vi "Begin.vi"(8 "error in":errorcluster) -> (0 "error out":errorcluster)   [LabVIEW 2016]
doc: "Called before other user functions, this VI is expected to open initial I/O refnums, load in file data, and do all program initialization. Notice that the <B>error out</B> terminal is simply used for data flow. Wiring it to other structures or subVIs ensures that this VI runs first."
uses:
  <vilib>/Rock Robotics/SystemInterfaces/DIO/FPGA_DIOPWMChannel.ctl
  <vilib>/Rock Robotics/WPI/SafetyOutput/WPI_SafetyOutputConfigMenu.ctl
  <vilib>/Rock Robotics/WPI/DriverStation/WPI_DriverStationRobotMode2.ctl
  <vilib>/Rock Robotics/WPI/Joystick/WPI_JoystickDeviceEnum.ctl
  <vilib>/Rock Robotics/SystemInterfaces/DIO/FPGA_DIOChannel.ctl
  <vilib>/Rock Robotics/SystemInterfaces/AI/FPGA_AIChannel.ctl
  <vilib>/Rock Robotics/WPI/RobotDrive/WPI_RobotDriveOpen2MotorWithVictorSP.vi
  Robot Global Data.vi
  <vilib>/Rock Robotics/Network Tables/NT Write String Array.vi
  <vilib>/Rock Robotics/WPI/MotorControl/WPI_MotorControlOpen VictorSP.vi
  <vilib>/Rock Robotics/WPI/Switch/WPI_SwitchOpenLimit.vi
  <vilib>/Rock Robotics/WPI/Counter/WPI_CounterDigitalInputToDigitalSource.vi
  <vilib>/Rock Robotics/WPI/Counter/WPI_CounterOpen UpDown Mode.vi
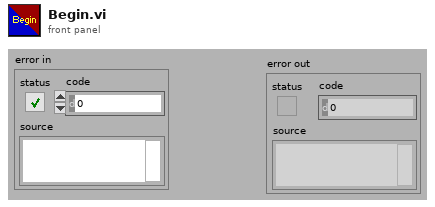
[diagram p1: front panel]
types:
  T1 = typedef "FPGA_DIOChannel.ctl" = enum8{"DIO 0", "DIO 1", "DIO 2", "DIO 3", "DIO 4", "DIO 5", "DIO 6", "DIO 7", "DIO 8", "DIO 9", "DIO MXP 0", "DIO MXP 1", "DIO MXP 2", "DIO MXP 3", "DIO MXP 4", "DIO MXP 5", "DIO MXP 6", "DIO MXP 7", "DIO MXP 8", "DIO MXP 9", "DIO MXP 10", "DIO MXP 11", "DIO MXP 12", "DIO MXP 13", "DIO MXP 14", "DIO MXP 15", "SPI Port CS1", "SPI Port CS2", "SPI Port CS3", "SPI Port MISO", "SPI Port MOSI", "Invalid"}
  T2 = typedef "FPGA_AIChannel.ctl" = enum8{"AI 0", "AI 1", "AI 2", "AI 3", "AI MXP 0", "AI MXP 1", "AI MXP 2", "AI MXP 3", "Invalid"}
  T3 = typedef "FPGA_DIOPWMChannel.ctl" = enum8{"PWM 0", "PWM 1", "PWM 2", "PWM 3", "PWM 4", "PWM 5", "PWM 6", "PWM 7", "PWM 8", "PWM 9", "PWM MXP 0", "PWM MXP 1", "PWM MXP 2", "PWM MXP 3", "PWM MXP 4", "PWM MXP 5", "PWM MXP 6", "PWM MXP 7", "PWM MXP 8", "PWM MXP 9", "Invalid"}
  T4 = typedef "WPI_JoystickDeviceEnum.ctl" = enum16{"USB 0", "USB 1", "USB 2", "USB 3", "USB 4", "USB 5"}
  T5 = typedef "WPI_DriverStationRobotMode2.ctl" = enum16{"Autonomous Disabled", "Autonomous Enabled", "Teleop Disabled", "Teleop Enabled", "Disconnected", "Finish", "Test Disabled", "Test Enabled", "Emergency Stopped"}
  T6 = typedef "WPI_SafetyOutputConfigMenu.ctl" = enum16{"Enable", "Disable"}
  T7 = typedef "WPI_MotorControlDeviceRef.ctl" = cluster{"DeviceStatus":errorcluster, "Type":T8, "PWM":cluster{"PWM Channel":T3, "DeadBand":T9}, "CAN":cluster{"Device Number":u8, "SetOutput VI Ref":variant, "GetOutput VI Ref":variant, "Enable VI Ref":variant, "Disable VI Ref":variant, "Data":variant}, "Invert":bool}
  T8 = typedef "WPI_MotorControlType.ctl" = enum16{"PWM", "CAN"}
  T9 = typedef "WPI_PWMDeadband.ctl" = cluster{"Name":string, "maxPositivePwm":i32, "minPositivePwm":i32, "centerPwm":i32, "maxNegativePwm":i32, "minNegativePwm":i32, "angularRange":u16}
  T10 = typedef "WPI_RobotDriveDevRef.ctl" = cluster{"DevStatus":errorcluster, "Motors[]":T7[], "Square Inputs":bool, "Max Output":dbl}
  T11 = typedef "WPI_JoystickDevRef.ctl" = cluster{"Device":T4}
  T12 = typedef "WPI_ServoDeviceRef.ctl" = cluster{"DeviceStatus":errorcluster, "PWM Channel":T3, "DeadBand":T9}
  T13 = typedef "WPI_SwitchDevRef.ctl" = cluster{"DevStatus":errorcluster, "DIO Channel":T1, "CntIndex":T14, "Normally Closed":bool}
  T14 = typedef "FPGA_CounterCtrSystemIndex.ctl" = enum8{"Ctr 0", "Ctr 1", "Ctr 2", "Ctr 3", "Ctr 4", "Ctr 5", "Ctr 6", "Ctr 7", "Invalid"}
  T15 = typedef "WPI_PotentiometerDevRef.ctl" = cluster{"DevStatus":errorcluster, "Analog Channel":T2, "Invert Output":bool}
  T16 = typedef "WPI_DigitalInputDevRef.ctl" = cluster{"DevStatus":errorcluster, "DIO Channel":T1}
  T17 = typedef "FPGA_CounterEncoderSourceConvertionLVSourceType.ctl" = cluster{"DevStatus":errorcluster, "AnalogTriggerMode?":bool, "DigitalMode":cluster{"DIO Channel":T18}, "AnalogTriggerMode":cluster{"AnalogTriggerIndex":T19, "OutputType":T20}}
  T18 = typedef "FPGA_DIODigitalSourceChannel.ctl" = enum8{"DIO 0", "DIO 1", "DIO 2", "DIO 3", "DIO 4", "DIO 5", "DIO 6", "DIO 7", "DIO 8", "DIO 9", "DIO MXP 0", "DIO MXP 1", "DIO MXP 2", "DIO MXP 3", "DIO MXP 4", "DIO MXP 5", "DIO MXP 6", "DIO MXP 7", "DIO MXP 8", "DIO MXP 9", "DIO MXP 10", "DIO MXP 11", "DIO MXP 12", "DIO MXP 13", "DIO MXP 14", "DIO MXP 15", "Disabled"}
  T19 = typedef "FPGA_AnalogTriggerIndex.ctl" = enum8{"Trig 0", "Trig 1", "Trig 2", "Trig 3", "Trig 4", "Trig 5", "Trig 6", "Trig 7", "Invalid"}
  T20 = typedef "FPGA_AnalogTriggerOutType.ctl" = enum16{"InWindow", "TriggerState", "Rising", "Falling"}
  T21 = typedef "WPI_CounterDevRef.ctl" = cluster{"DevStatus":errorcluster, "CntIndex":T14}
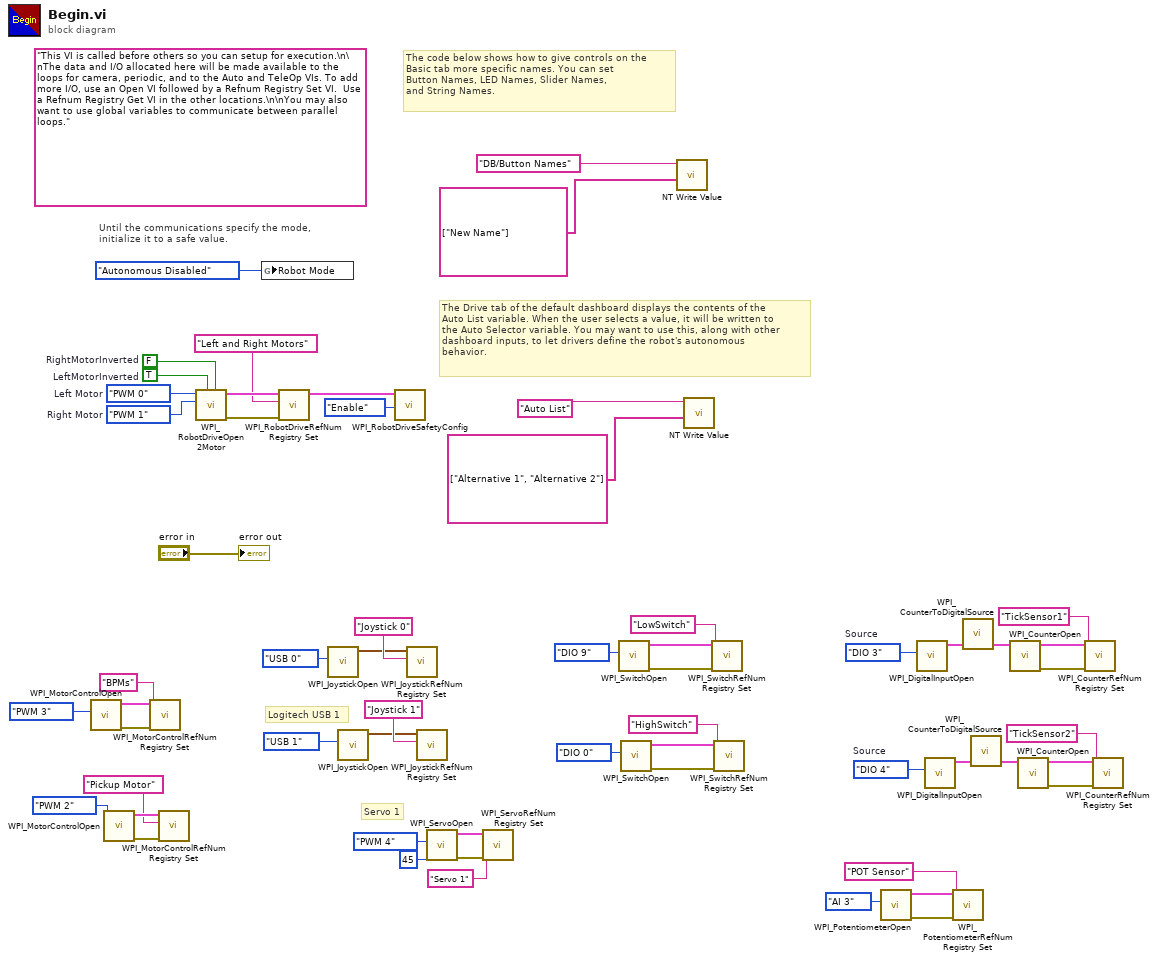
[diagram p0: block diagram]
diagram:
  w5 = FPGA_DIOChannel."DIO 4"  # Source
  w11 = FPGA_DIOChannel."DIO 3"  # Source
  (unwired) "This VI is called before others so you can setup for execution.\n\nThe data and I/O allocated here will be made available to the loops for camera, periodic, and to the Auto and TeleOp VIs. To add more I/O, use an Open VI followed by a Refnum Registry Set VI.  Use a Refnum Registry Get VI in the other locations.\n\nYou may also want to use global variables to communicate between parallel loops."
  w52 = FPGA_DIOPWMChannel."PWM 1"  # Right Motor
  w53 = FPGA_DIOPWMChannel."PWM 0"  # Left Motor
  w57 = TRUE  # LeftMotorInverted
  w58 = FALSE  # RightMotorInverted
  # "Logitech USB 1"
  # "Servo 1"
  # "The Drive tab of the default dashboard displays the contents of the\nAuto List variable. When the user selects a value, it will be written to\nthe Auto Selector variable. You may want to use this, along with other\ndashboard inputs, to let drivers define the robot's autonomous\nbehavior."
  # "The code below shows how to give controls on the\nBasic tab more specific names. You can set\nButton Names, LED Names, Slider Names,\nand String Names."
  # "Until the communications specify the mode,\ninitialize it to a safe value."
  n1 = call-poly <vilib>:"WPI_MotorControlOpen.vi"("PWM Channel"=FPGA_DIOPWMChannel."PWM 3") -> ("error out"=w32:errorcluster, "MotorControlDeviceRef"=w31:T7)  [unwired: 9 in]
  n2 = call-poly <vilib>:"WPI_MotorControlOpen.vi"("PWM Channel"=FPGA_DIOPWMChannel."PWM 2") -> ("error out"=w40:errorcluster, "MotorControlDeviceRef"=w39:T7)  [unwired: 9 in]
  n3 = call <vilib>:"WPI_MotorControlRefNum Registry Set.vi"("error in (no error)"=w32, "refnum name"="BPMs", "MotorControlDevRef"=w31) -> ()  [unwired: 7 in, 2 out]
  n4 = call <vilib>:"WPI_MotorControlRefNum Registry Set.vi"("error in (no error)"=w40, "refnum name"="Pickup Motor", "MotorControlDevRef"=w39) -> ()  [unwired: 7 in, 2 out]
  n5 = call-poly <vilib>:"WPI_RobotDriveOpen2Motor.vi"("Right Motor Inverted"=w58, "Left Motor Inverted"=w57, "Right Motor"=w52, "Left Motor"=w53) -> ("error out"=w54:errorcluster, "RobotDriveDevRef"=w56:T10)  [unwired: 1 in, 5 out]
  n6 = global write "Robot Global Data.vi" "Robot Mode"(WPI_DriverStationRobotMode2."Autonomous Disabled" ("Robot Mode")) -> ()
  n7 = call <vilib>:"WPI_RobotDriveRefNum Registry Set.vi"("error in (no error)"=w54, "refnum name"="Left and Right Motors", "RobotDriveDevRef"=w56) -> ("RobotDriveDevRef"=w51:T10)  [unwired: 1 in, 7 out]
  n8 = call <vilib>:"WPI_JoystickOpen.vi"("JoystickDevice"=WPI_JoystickDeviceEnum."USB 0") -> ("JoystickDevRef"=w47:T11)  [unwired: 10 in]
  n9 = call <vilib>:"WPI_JoystickOpen.vi"("JoystickDevice"=WPI_JoystickDeviceEnum."USB 1") -> ("JoystickDevRef"=w35:T11)  [unwired: 10 in]
  n10 = call <vilib>:"WPI_RobotDriveSafetyConfig.vi"("mode"=WPI_SafetyOutputConfigMenu."Enable", "RobotDriveDevRef"=w51) -> ()  [unwired: 8 in, 2 out]
  n11 = call <vilib>:"WPI_JoystickRefNum Registry Set.vi"("refnum name"="Joystick 0", "JoystickDevRef"=w47) -> ()  [unwired: 8 in, 2 out]
  n12 = call <vilib>:"WPI_JoystickRefNum Registry Set.vi"("refnum name"="Joystick 1", "JoystickDevRef"=w35) -> ()  [unwired: 8 in, 2 out]
  n13 = call <vilib>:"WPI_ServoOpen.vi"("Angular Range"=u16 45, "PWM Channel"=FPGA_DIOPWMChannel."PWM 4") -> ("error out"=w27:errorcluster, "ServoDeviceRef"=w26:T12)  [unwired: 8 in]
  n14 = call <vilib>:"WPI_ServoRefNum Registry Set.vi"("error in (no error)"=w27, "refnum name"="Servo 1", "ServoDeviceRef"=w26) -> ()  [unwired: 7 in, 2 out]
  n15 = call-poly <vilib>:"WPI_SwitchOpen.vi"("DIO Channel"=FPGA_DIOChannel."DIO 9") -> ("error out"=w24:errorcluster, "SwitchDevRef"=w23:T13)  [unwired: 9 in]
  n16 = call-poly <vilib>:"WPI_SwitchOpen.vi"("DIO Channel"=FPGA_DIOChannel."DIO 0") -> ("error out"=w20:errorcluster, "SwitchDevRef"=w19:T13)  [unwired: 9 in]
  n17 = call-poly <vilib>:"NT Write Value.vi"("String Array"=string[] ["New Name"], "Name"="DB/Button Names") -> ()  [unwired: 9 in, 1 out]
  n18 = call-poly <vilib>:"NT Write Value.vi"("String Array"=string[] ["Alternative 1", "Alternative 2"], "Name"="Auto List") -> ()  [unwired: 9 in, 1 out]
  n19 = call <vilib>:"WPI_SwitchRefNum Registry Set.vi"("error in (no error)"=w24, "refnum name"="LowSwitch", "SwitchDevRef"=w23) -> ()  [unwired: 7 in, 2 out]
  n20 = call <vilib>:"WPI_SwitchRefNum Registry Set.vi"("error in (no error)"=w20, "refnum name"="HighSwitch", "SwitchDevRef"=w19) -> ()  [unwired: 7 in, 2 out]
  n21 = call <vilib>:"WPI_PotentiometerOpen.vi"("Analog Channel"=FPGA_AIChannel."AI 3") -> ("error out"=w16:errorcluster, "PotDevRef"=w15:T15)  [unwired: 9 in]
  n22 = call <vilib>:"WPI_DigitalInputOpen.vi"("DIO Channel"=w11) -> ("DigitalInputDevRef"=w10:T16)  [unwired: 1 in, 9 out]
  n23 = call <vilib>:"WPI_DigitalInputOpen.vi"("DIO Channel"=w5) -> ("DigitalInputDevRef"=w4:T16)  [unwired: 1 in, 9 out]
  n24 = call <vilib>:"WPI_PotentiometerRefNum Registry Set.vi"("error in (no error)"=w16, "refnum name"="POT Sensor", "PotDevRef"=w15) -> ()  [unwired: 7 in, 2 out]
  n25 = call-poly <vilib>:"WPI_CounterToDigitalSource.vi"("DigitalInputDevRef"=w10) -> ("Digital Source"=w12:T17)  [unwired: 6 out]
  n26 = call-poly <vilib>:"WPI_CounterToDigitalSource.vi"("DigitalInputDevRef"=w4) -> ("Digital Source"=w6:T17)  [unwired: 6 out]
  n27 = call-poly <vilib>:"WPI_CounterOpen.vi"("Up Source"=w12) -> ("error out"=w9:errorcluster, "CounterDevRef"=w8:T21)  [unwired: 6 in, 3 out]
  n28 = call-poly <vilib>:"WPI_CounterOpen.vi"("Up Source"=w6) -> ("error out"=w3:errorcluster, "CounterDevRef"=w2:T21)  [unwired: 6 in, 3 out]
  n29 = call <vilib>:"WPI_CounterRefNum Registry Set.vi"("error in (no error)"=w9, "refnum name"="TickSensor1", "CounterDevRef"=w8) -> ()  [unwired: 7 in, 2 out]
  n30 = call <vilib>:"WPI_CounterRefNum Registry Set.vi"("error in (no error)"=w3, "refnum name"="TickSensor2", "CounterDevRef"=w2) -> ()  [unwired: 7 in, 2 out]
  "error out" <- "error in"
